vi "Get Buffer Address.vi"(11 "Buffer in":refnum<class "Buffer.lvclass">) -> (2 "buffer address":u64 format="%016x", 3 "Buffer out":refnum<class "Buffer.lvclass">)   [LabVIEW 2017, in "DSF Core.lvlib" / "Buffer.lvclass"]
uses:
  Buffer.lvclass
  C:/Git/DSF/LabVIEW-Memory/Source/Classes/Pointer/Pointer.lvclass
  LabVIEW-Memory/Source/Classes/Pointer/Pointer.lvclass
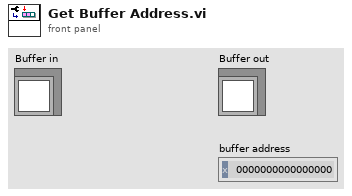
[diagram p1: front panel]
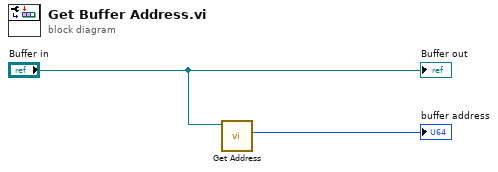
[diagram p0: block diagram]
diagram:
  n1 = call "Get Address.vi"("Pointer in"="Buffer in") -> ("address"=→"buffer address":u64)  [unwired: 9 in, 1 out]
  "Buffer out" <- "Buffer in"
